vi "Run Installer.vi"(8 "error in":errorcluster, 11 "installer path in":path) -> (0 "error out":errorcluster, 3 "installer path out":path)   [LabVIEW 2018]
uses:
  <vilib>/Utility/config.llb/Write Key (I32).vi
  <vilib>/Utility/config.llb/NI_LVConfig.lvlib
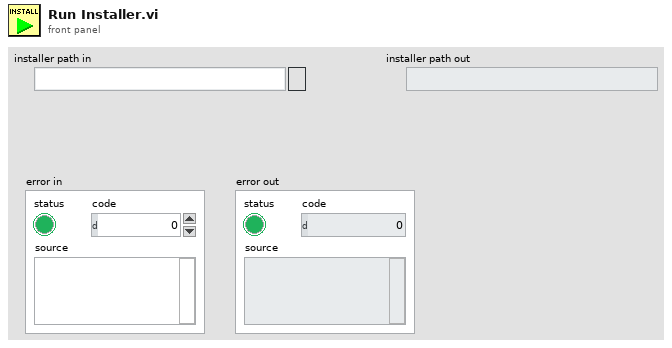
[diagram p1: front panel]
types:
  T1 = typedef "NI_LVConfig.lvlib/Config Data RefNum.ctl" = refnum<k1>
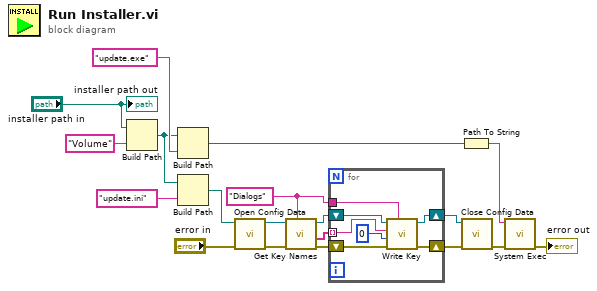
[diagram p0: block diagram]
diagram:
  w2 = "Dialogs" ("section")
  n1 = Build Path(base path="installer path in", name or relative path="Volume") -> (appended path=w13:path)
  n2 = Build Path(base path=w13, name or relative path="update.exe") -> (appended path=w16:path)
  n3 = Build Path(base path=w13, name or relative path="update.ini") -> (appended path=w12:path)
  n4 = call <vilib>:"Open Config Data.vi"("error in (no error)"="error in", "configuration file path"=w12) -> ("error out"=w6:errorcluster, "refnum"=w9:T1)  [unwired: 7 in, 1 out]
  n5 = call <vilib>:"Get Key Names.vi"("section"=w2, "error in (no error)"=w6, "refnum"=w9) -> ("error out"=w7:errorcluster, "key names"=w5:string[], "refnum out"=w8:T1)  [unwired: 5 in, 1 out]
  n6 = for {
    shift-right: [w25] -> w11
    shift-left: w8 -> [w26]
    shift-right: [w24] -> w10
    shift-left: w7 -> [w23]
    tunnel: w5 -> [w22] mode=indexing
    tunnel: w2 -> [w21]
    n7 = call-poly <vilib>:"Write Key.vi"("section"=w21, "error in (no error)"=w23, "value"=0, "key"=w22, "refnum"=w26) -> ("error out"=w24:errorcluster, "refnum out"=w25:T1)  [unwired: 4 in, 1 out]
  }
  n8 = Path To String(path=w16) -> (string=w15:string)
  n9 = call <vilib>:"Close Config Data.vi"("error in (no error)"=w10, "refnum"=w11) -> ("error out"=w3:errorcluster)  [unwired: 8 in, 1 out]
  n10 = call <vilib>:"System Exec.vi"("error in (no error)"=w3, "command line"=w15) -> ("error out"=→"error out":errorcluster)  [unwired: 6 in, 3 out]
  "installer path out" <- "installer path in"
